vi "RT_TVA_DATA_v2.vi"(11 "TVA_Data":u64[](array[numeric])) -> (0 "Yaw stream":dbl, 1 "Pitch stream":dbl, 2 "Yaw Angle":dbl(knob) scale=-3.0..3.0, 3 "Pitch Angle":dbl(knob) scale=-3.0..3.0, 4 "Data CRC Fault":bool, 5 "Yaw desired":dbl, 6 "Address CRC Fault":bool, 7 "Pitch desired":dbl)   [LabVIEW 2017]
panel:
  out "Roll Angle":dbl
  out "Roll Rate":dbl
  out "element":u64 format="%x"
  out "element 4":u64 format="%x"
  out "element 3":u64 format="%x"
  out "element 2":u64 format="%x"
  out "Dest address":u8
  out "Souce address":u8
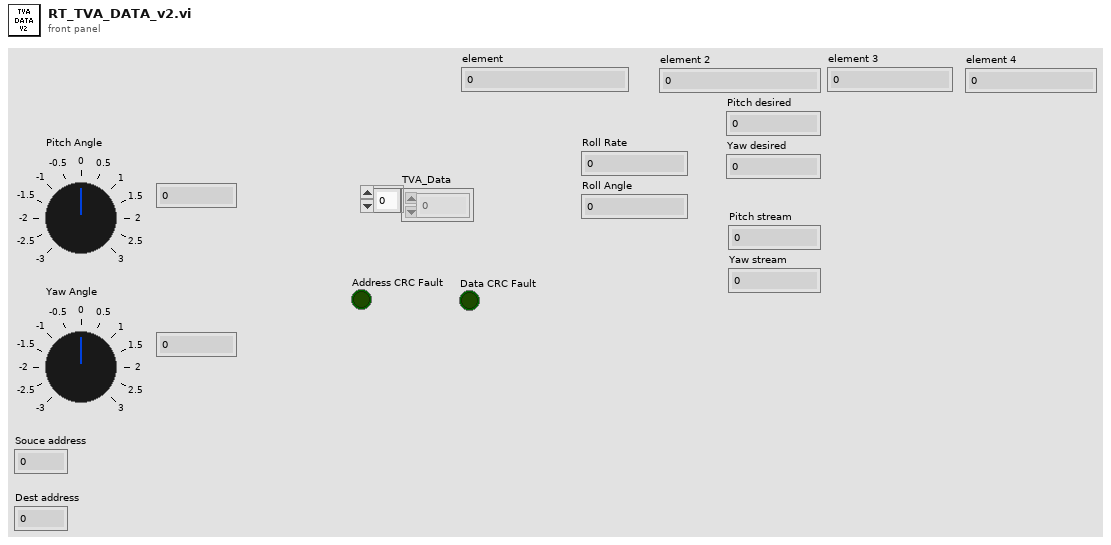
[diagram p1: front panel]
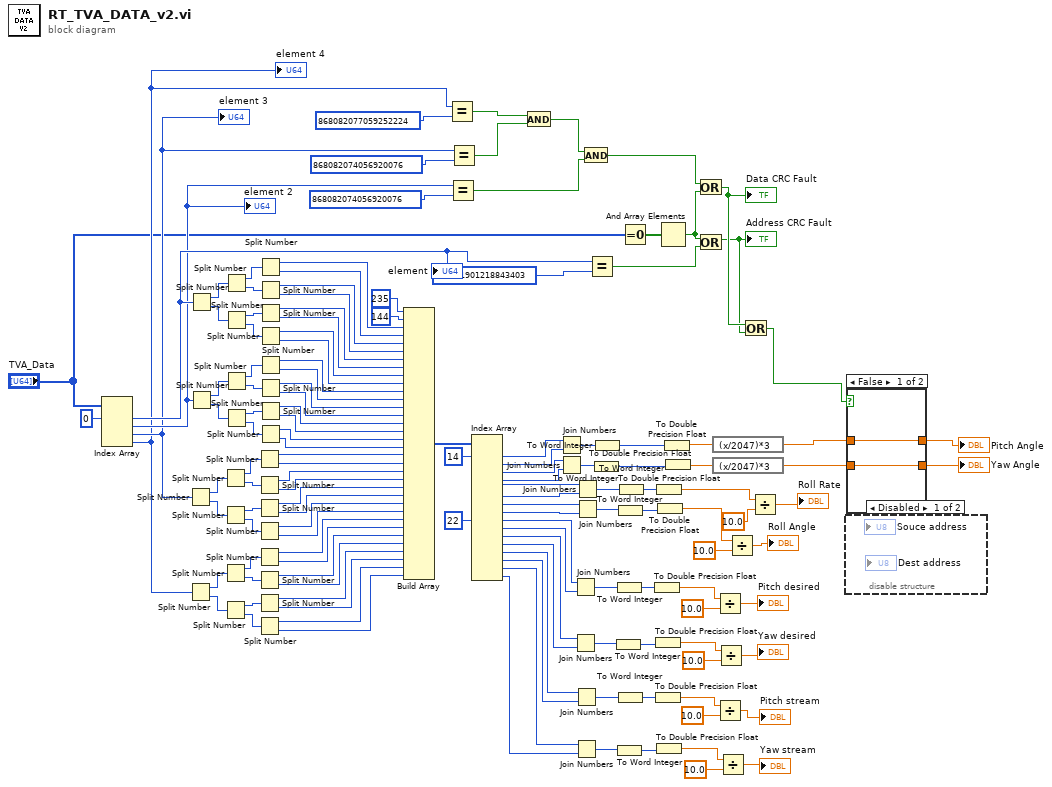
[diagram p0: block diagram]
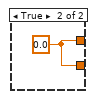
[diagram p3: hidden frame]
diagram:
  n1 = Index Array(array="TVA_Data", index #1=0 ("index")) -> (element #1=w70:u64, element #2=w67:u64, element #3=w65:u64, element #4=w63:u64)  [unwired: 3 in]
  "element 2" <- w67
  "element 3" <- w65
  "element 4" <- w63
  "element" <- w70
  n2 = Split Number(x=w65) -> (hi(x)=w86:u32, lo(x)=w87:u32)
  n3 = Split Number(x=w63) -> (hi(x)=w97:u32, lo(x)=w96:u32)
  n4 = Split Number(x=w70) -> (hi(x)=w74:u32, lo(x)=w75:u32)
  n5 = Split Number(x=w67) -> (hi(x)=w85:u32, lo(x)=w84:u32)
  n6 = Split Number(x=w86) -> (hi(x)=w88:u16, lo(x)=w89:u16)
  n7 = Split Number(x=w87) -> (hi(x)=w90:u16, lo(x)=w91:u16)
  n8 = Split Number(x=w97) -> (hi(x)=w95:u16, lo(x)=w94:u16)
  n9 = Split Number(x=w96) -> (hi(x)=w93:u16, lo(x)=w92:u16)
  n10 = Split Number(x=w74) -> (hi(x)=w76:u16, lo(x)=w77:u16)
  n11 = Split Number(x=w75) -> (hi(x)=w78:u16, lo(x)=w79:u16)
  n12 = Split Number(x=w85) -> (hi(x)=w83:u16, lo(x)=w82:u16)
  n13 = Split Number(x=w84) -> (hi(x)=w81:u16, lo(x)=w80:u16)
  n14 = Split Number(x=w88) -> (hi(x)=w113:u8, lo(x)=w114:u8)
  n15 = Split Number(x=w89) -> (hi(x)=w115:u8, lo(x)=w116:u8)
  n16 = Split Number(x=w90) -> (hi(x)=w117:u8, lo(x)=w118:u8)
  n17 = Split Number(x=w91) -> (hi(x)=w119:u8, lo(x)=w120:u8)
  n18 = Split Number(x=w95) -> (hi(x)=w121:u8, lo(x)=w122:u8)
  n19 = Split Number(x=w94) -> (hi(x)=w123:u8, lo(x)=w124:u8)
  n20 = Split Number(x=w93) -> (hi(x)=w125:u8, lo(x)=w126:u8)
  n21 = Split Number(x=w92) -> (hi(x)=w137:u8, lo(x)=w138:u8)
  n22 = Split Number(x=w76) -> (hi(x)=w98:u8, lo(x)=w99:u8)
  n23 = Split Number(x=w77) -> (hi(x)=w100:u8, lo(x)=w101:u8)
  n24 = Split Number(x=w78) -> (hi(x)=w102:u8, lo(x)=w103:u8)
  n25 = Split Number(x=w79) -> (hi(x)=w104:u8, lo(x)=w105:u8)
  n26 = Split Number(x=w83) -> (hi(x)=w71:u8, lo(x)=w106:u8)
  n27 = Split Number(x=w82) -> (hi(x)=w107:u8, lo(x)=w108:u8)
  n28 = Split Number(x=w81) -> (hi(x)=w109:u8, lo(x)=w110:u8)
  n29 = Split Number(x=w80) -> (hi(x)=w111:u8, lo(x)=w112:u8)
  n30 = Build Array(u8 235 ("x"), u8 144 ("x"), w98, w99, w100, w101, w102, w103, w104, w105, w71, w106, w107, w108, w109, w110, w111, w112, w113, w114, w115, w116, w117, w118, w119, w120, w121, w122, w123, w124, w125, w126, w137, w138) -> (w127:u8[])
  n31 = Equal?(x=w63, y=u64 868082077059252224) -> (x = y?=w62:bool)
  n32 = Equal?(x=w67, y=u64 868082074056920076) -> (x = y?=w59:bool)
  n33 = Equal?(x=w65, y=u64 868082074056920076) -> (x = y?=w61:bool)
  n34 = Index Array(array=w127, index #1=14 ("index"), index #9=22 ("index")) -> (element #1=w131:u8, element #2=w132:u8, element #3=w133:u8, element #4=w134:u8, element #5=w47:u8, element #6=w46:u8, element #7=w45:u8, element #8=w44:u8, element #9=w20:u8, element #10=w19:u8, element #11=w18:u8, element #12=w17:u8, element #13=w16:u8, element #14=w15:u8, element #15=w14:u8, element #16=w13:u8)  [unwired: 14 in]
  n35 = And(x=w62, y=w61) -> (x .and. y?=w60:bool)
  n36 = Join Numbers(hi=w131, lo=w132) -> ((hi.lo)=w37:u16)
  n37 = Join Numbers(hi=w133, lo=w134) -> ((hi.lo)=w35:u16)
  n38 = Join Numbers(hi=w20, lo=w19) -> ((hi.lo)=w25:u16)
  n39 = Join Numbers(hi=w18, lo=w17) -> ((hi.lo)=w26:u16)
  n40 = Join Numbers(hi=w16, lo=w15) -> ((hi.lo)=w24:u16)
  n41 = Join Numbers(hi=w14, lo=w13) -> ((hi.lo)=w23:u16)
  n42 = Join Numbers(hi=w47, lo=w46) -> ((hi.lo)=w33:u16)
  n43 = Join Numbers(hi=w45, lo=w44) -> ((hi.lo)=w32:u16)
  n44 = And(x=w60, y=w59) -> (x .and. y?=w55:bool)
  n45 = Equal?(x=w70, y=u64 795741901218843403) -> (x = y?=w69:bool)
  n46 = To Word Integer(number=w35) -> (16bit integer=w34:i16)
  n47 = To Word Integer(number=w37) -> (16bit integer=w36:i16)
  n48 = To Word Integer(number=w26) -> (16bit integer=w27:i16)
  n49 = To Word Integer(number=w25) -> (16bit integer=w28:i16)
  n50 = To Word Integer(number=w23) -> (16bit integer=w22:i16)
  n51 = To Word Integer(number=w32) -> (16bit integer=w31:i16)
  n52 = To Word Integer(number=w24) -> (16bit integer=w21:i16)
  n53 = To Word Integer(number=w33) -> (16bit integer=w30:i16)
  n54 = Equal To 0?(x="TVA_Data") -> (x = 0?=w57:bool[])
  n55 = To Double Precision Float(number=w28) -> (double precision float=w11:dbl)
  n56 = To Double Precision Float(number=w27) -> (double precision float=w7:dbl)
  n57 = To Double Precision Float(number=w21) -> (double precision float=w6:dbl)
  n58 = To Double Precision Float(number=w30) -> (double precision float=w38:dbl)
  n59 = To Double Precision Float(number=w22) -> (double precision float=w5:dbl)
  n60 = To Double Precision Float(number=w31) -> (double precision float=w40:dbl)
  n61 = And Array Elements(Boolean array=w57) -> (logical AND=w56:bool)
  n62 = To Double Precision Float(number=w36) -> (double precision float=w136:dbl)
  n63 = To Double Precision Float(number=w34) -> (double precision float=w135:dbl)
  n64 = Or(x=w55, y=w56) -> (x .or. y?=w54:bool)
  "Data CRC Fault" <- w54
  n65 = Or(x=w56, y=w69) -> (x .or. y?=w53:bool)
  "Address CRC Fault" <- w53
  n66 = expression code="(x/2047)*3"(w136) -> (w49:dbl)
  n67 = expression code="(x/2047)*3"(w135) -> (w48:dbl)
  n68 = Divide(x=w11, y=10.0) -> (x/y=→"Pitch desired":dbl)
  n69 = Divide(x=w6, y=10.0) -> (x/y=→"Pitch stream":dbl)
  n70 = Divide(x=w7, y=10.0) -> (x/y=→"Yaw desired":dbl)
  n71 = Divide(x=w5, y=10.0) -> (x/y=→"Yaw stream":dbl)
  n72 = Divide(x=w40, y=10.0) -> (x/y=→"Roll Angle":dbl)
  n73 = Or(x=w54, y=w53) -> (x .or. y?=w52:bool)
  n74 = Divide(x=w38, y=10.0) -> (x/y=→"Roll Rate":dbl)
  n75 = disable-structure shown="Disabled" {
    frame Disabled {
    }
    frame Enabled {
    }
  }
  n76 = case shown="False" w52 {
    tunnel: [w140 w141] -> w51
    tunnel: [w139 w141] -> w50
    tunnel: w49 -> [w140 _]
    tunnel: w48 -> [w139 _]
    frame False {
    }
    frame True {
      w141 = 0.0
    }
  }
  "Yaw Angle" <- w50
  "Pitch Angle" <- w51
